vi "PH_HamamatsuCamera.PC Write PSDB.vi"(0 "i ref in":refnum<vi>, 5 "error IO":errorcluster) -> (14 "i ref out":refnum<vi>, 19 "error out":errorcluster)   [LabVIEW 2014, in "PH_HamamatsuCamera.lvlib"]
doc: "This is the proc case which writes data to the PHELIX shot data base."
uses:
  PH_HamamatsuCamera.lvlib
  PH_Basics/PH_PSDBWriter/PH_PSDBWriter.lvlib
  PH_Basics/PH_Cam_BaseClass/PH_Cam_BaseClass.lvlib
  PH_Basics/PH_StatusHandler/PH_StatusHandler.lvlib
panel:
  in  "Mode":u32(ring)=1 items=["Internal"=1, "External Edge"=2, "External Level"=4, "Software"=32, "Fast Repetition"=64, "TDI"=128, "Trigger Start"=512, "Sync Readout"=1024]
  in  "Polarity":u32(ring)=1 items=["Negative"=1, "Positive"=2]
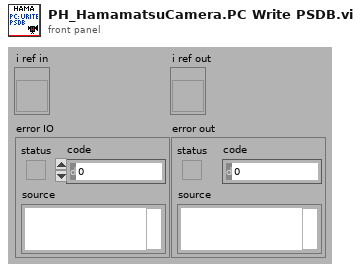
[diagram p1: front panel]
types:
  T1 = typedef "PH_HamamatsuCamera.lvlib/PH_HamamatsuCamera.i attribute.ctl" = cluster{"Gui Refs":cluster{"Camera Details":refnum<vi>, "ROI":refnum<vi>, "Set ROI to Maximum":refnum<vi>, "Trigger Parameters":refnum<vi>, "Brightness":refnum<vi>, "Shutter":refnum<vi>, "Gain":refnum<vi>, "Trigger Timeout":refnum<vi>, "Trigger Polarity":refnum<vi>, "Trigger Mode":refnum<vi>, "Parameters":refnum<vi>, "Set Cam Parameter":refnum<vi>, "Parameter to set":refnum<vi>, "Value to set":refnum<vi>}, "Cam":cluster{"Handle":i32, "Details":cluster{"Model":string, "Camera ID":string, "Firmware":string}, "Buffer Info":cluster{"height":u32, "width":u32, "datatype":u32}}, "H Offset":cluster{"Value":i32, "Minimum":i32, "Maximum":i32, "Increment":i32}, "V Offset":cluster{"Value":i32, "Minimum":i32, "Maximum":i32, "Increment":i32}, "H Width":cluster{"Value":i32, "Minimum":i32, "Maximum":i32, "Increment":i32}, "V Width":cluster{"Value":i32, "Minimum":i32, "Maximum":i32, "Increment":i32}, "Trigger Parameters":T2, "Trigger Timeout":u32, "Parameters":T3[], "Indicees Cam Parameters":cluster{"Brightness":i32, "Shutter":i32, "Gain":i32}, "Wanted Values":cluster{"Trigger Settings":T2[], "ROI":T4[], "Parameter":cluster{"Name":string, "Value":dbl}[]}}
  T2 = typedef "PH_HamamatsuCamera.lvlib/PH_HamamatsuCamera.Trigger Parameter.ctl" = cluster{"Mode":u32, "Polarity":u32, "Times":u32, "Delay":dbl}
  T3 = typedef "PH_HamamatsuCamera.lvlib/PH_HamamatsuCamera.Parameter Set.ctl" = cluster{"Parameter":string, "Value":dbl, "Writable":bool, "Range":cluster{"min":dbl, "max":dbl, "step":dbl}, "Default":dbl, "Value Names":cluster{"Name":string, "Value":dbl}[], "Text Values":bool}
  T4 = typedef "PH_HamamatsuCamera.lvlib/PH_HamamatsuCamera.ROI.ctl" = cluster{"Horizontal Offset":i32, "Vertical Offset":i32, "Horizontal Width":i32, "Vertical Width":i32}
  T5 = typedef "LVStringsAndValuesArrayTypeDef_U32.ctl" = cluster{"String":string, "Value":u32}[]
  T6 = typedef "PH_Cam_BaseClass.lvlib/PH_Cam_BaseClass.Settings.ctl" = cluster{"Cam ID":string, "Gain":dbl, "Brightness":dbl, "Shutter":dbl, "Mode":i32}
  T7 = typedef "PH_StatusHandler.lvlib/PH_StatusHandler.Status.ctl" = i16
  T8 = typedef "PH_Cam_BaseClass.lvlib/PH_Cam_BaseClass.i attribute.ctl" = cluster{"Gui Refs":T9, "Cam":cluster{"Source Notifier":refnum<notifier>, "Error":errorcluster, "Camera ID":string}, "Images":cluster{"Cam":T10, "Operation":T10, "PSDB":T10}, "Window Image":cluster{"Indicate Image":bool, "Window No.":i32, "Scale Facor":dbl, "Center Cross":bool, "Subtract Backgr":bool, "CoG":bool, "Color Palette":cluster{"Red":u8, "Green":u8, "Blue":u8}[], "Image On":bool}, "Default Prdc Int":i32, "Performance":cluster{"on":bool, "Timestamp Last Frame":i32}, "Histogram":cluster{"on":bool, "Mapping":bool}, "Save Image":cluster{"Save":bool, "File refnum":refnum<file>}, "Setting Service ID":i32, "Screen":cluster{"x-resolution":i16, "y-resolution":i16}, "On":bool, "Constructor finished":bool, "configured":bool}
  T9 = typedef "PH_Cam_BaseClass.lvlib/PH_Cam_BaseClass.GUI Refs.ctl" = cluster{"Frame Rate":refnum<vi>, "Get Frame Rate":refnum<vi>, "Show Image":refnum<vi>, "Get Histogram":refnum<vi>, "Mapping":refnum<vi>, "Histogram":refnum<vi>, "Center Cross":refnum<vi>, "Center of Gravity":refnum<vi>, "Scale Factor [%]":refnum<vi>, "Save Image":refnum<vi>, "Palette":refnum<vi>, "Subtract Background":refnum<vi>, "Cam Error":refnum<vi>, "On":refnum<vi>, "Cam List":refnum<vi>}
  T10 = typedef "IMAQ Image.ctl" = refnum<image>
  T11 = typedef "PH_PSDBWriter.lvlib/PH_PSDBWriter.Image dataset.ctl" = cluster{"name":string, "data":T10, "unit":string}
  T12 = typedef "PH_PSDBWriter.lvlib/PH_PSDBWriter.Numeric dataset.ctl" = cluster{"name":string, "data":dbl, "unit":string}
  T13 = typedef "PH_PSDBWriter.lvlib/PH_PSDBWriter.String dataset.ctl" = cluster{"name":string, "data":string, "unit":string}
  T14 = typedef "PH_PSDBWriter.lvlib/PH_PSDBWriter.PSDB Dataset.ctl" = cluster{"Version":i32, "2D data Input":T15[], "Boolean Input":T17[], "Image Input":T11[], "Numeric Input":T12[], "String Input":T13[]}
  T15 = typedef "PH_PSDBWriter.lvlib/PH_PSDBWriter.2D dataset.ctl" = cluster{"name":string, "data":dbl[][], "axis description":T16}
  T16 = typedef "PSDB.lvlib/PSDB_AxisDescription.ctl" = cluster{"x axis label":string, "y axis label":string, "x axis unit":string, "y axis unit":string}
  T17 = typedef "PH_PSDBWriter.lvlib/PH_PSDBWriter.Boolean dataset.ctl" = cluster{"name":string, "data":bool, "unit":string}
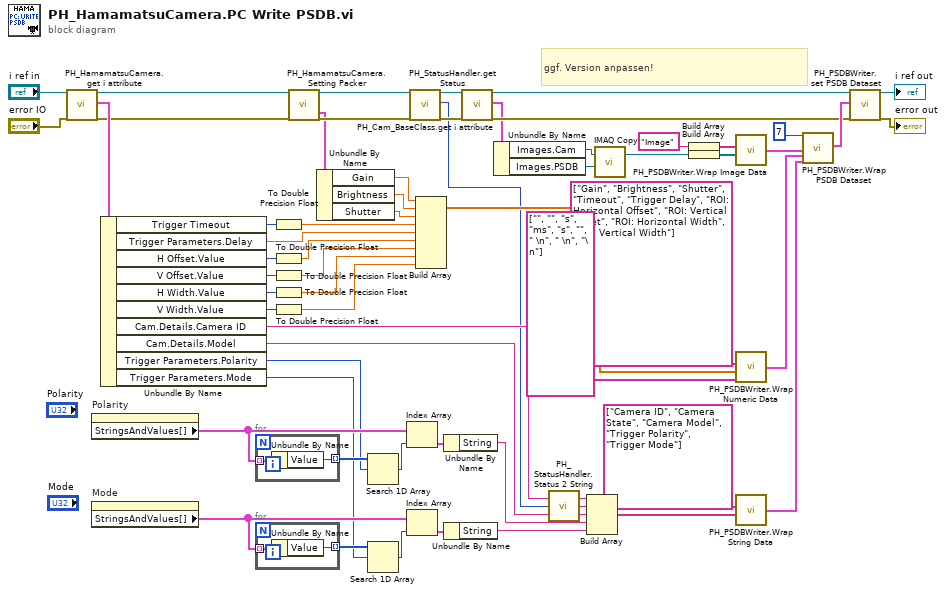
[diagram p0: block diagram]
diagram:
  # "ggf. Version anpassen!"
  n1 = call "PH_HamamatsuCamera.get i attribute.vi"("i ref in"="i ref in", "error in (no error)"="error IO") -> ("i ref out"=w38:refnum<vi>, "i attribute"=w57:T1, "error out"=w37:errorcluster)  [unwired: 15 in]
  n2 = property on="Polarity" class="Ring (strict)"() -> ("StringsAndValues[]"=w21:T5)  [unwired: 2 in, 2 out]
  n3 = property on="Mode" class="Ring (strict)"() -> ("StringsAndValues[]"=w15:T5)  [unwired: 2 in, 2 out]
  n4 = Unbundle By Name(w57) -> ("Trigger Timeout"=w58:u32, "Trigger Parameters.Delay"=w31:dbl, "H Offset.Value"=w12:i32, "V Offset.Value"=w11:i32, "H Width.Value"=w10:i32, "V Width.Value"=w9:i32, "Cam.Details.Camera ID"=w30:string, "Cam.Details.Model"=w55:string, "Trigger Parameters.Polarity"=w20:u32, "Trigger Parameters.Mode"=w14:u32)
  n5 = for {
    tunnel: w21 -> [w63] mode=indexing
    tunnel: [w62] -> w24 mode=indexing
    n6 = Unbundle By Name(w63) -> ("Value"=w62:u32)
  }
  n7 = for {
    tunnel: w15 -> [w65] mode=indexing
    tunnel: [w64] -> w18 mode=indexing
    n8 = Unbundle By Name(w65) -> ("Value"=w64:u32)
  }
  n9 = To Double Precision Float(number=w58) -> (double precision float=w59:dbl)
  n10 = To Double Precision Float(number=w12) -> (double precision float=w8:dbl)
  n11 = To Double Precision Float(number=w11) -> (double precision float=w7:dbl)
  n12 = To Double Precision Float(number=w10) -> (double precision float=w6:dbl)
  n13 = To Double Precision Float(number=w9) -> (double precision float=w5:dbl)
  n14 = call "PH_HamamatsuCamera.Setting Packer.vi"("i ref in"=w38, "error in (no error)"=w37) -> ("i ref out"=w3:refnum<vi>, "Cam Settings"=w35:T6, "error out"=w36:errorcluster)  [unwired: 15 in]
  n15 = Unbundle By Name(w35) -> ("Gain"=w34:dbl, "Brightness"=w33:dbl, "Shutter"=w32:dbl)
  n16 = Search 1D Array(1D array=w24, element=w20) -> (index of element=w23:i32)  [unwired: 1 in]
  n17 = Search 1D Array(1D array=w18, element=w14) -> (index of element=w17:i32)  [unwired: 1 in]
  n18 = Index Array(array=w21, index=w23) -> (element=w22:cluster{"String":string, "Value":u32})
  n19 = Index Array(array=w15, index=w17) -> (element=w16:cluster{"String":string, "Value":u32})
  n20 = call "PH_StatusHandler.get Status.vi"("VI in"=w3, "error in"=w36) -> ("VI out"=w2:refnum<vi>, "Status"=w1:T7, "error out"=w4:errorcluster)  [unwired: 15 in]
  n21 = Build Array(w34, w33, w32, w59, w31, w8, w7, w6, w5) -> (w47:dbl[])
  n22 = Unbundle By Name(w22) -> ("String"=w19:string)
  n23 = Unbundle By Name(w16) -> ("String"=w13:string)
  n24 = call "PH_Cam_BaseClass.get i attribute.vi"("i ref in"=w2, "error in (no error)"=w4) -> ("i ref out"=w28:refnum<vi>, "i attribute"=w27:T8, "error out"=w29:errorcluster)  [unwired: 15 in]
  n25 = Unbundle By Name(w27) -> ("Images.Cam"=w26:T10, "Images.PSDB"=w25:T10)
  n26 = call "PH_StatusHandler.Status 2 String.vi"("Status"=w1) -> ("Status as string"=w56:string)
  n27 = Build Array(w30, w56, w55, w19, w13) -> (w52:string[])
  n28 = call "IMAQ Copy"("Image Dst"=w25, "Image Src"=w26) -> ("Image Dst Out"=w42:T10)  [unwired: 4 in, 1 out]
  n29 = Build Array("Image" ("name")) -> (w39:string[])
  n30 = Build Array(w42) -> (w41:T10[])
  n31 = call "PH_PSDBWriter.Wrap Image Data.vi"("Data Arrray"=w41, "Name Array"=w39) -> ("PSDB Image Data Array"=w44:T11[])  [unwired: 2 in]
  n32 = call "PH_PSDBWriter.Wrap Numeric Data.vi"("Unit Array"=string[] ["", "", "s", "ms", "s", "", " \n", " \n", "\n"], "Data Array"=w47, "Name Array"=string[] ["Gain", "Brightness", "Shutter", "Timeout", "Trigger Delay", "ROI: Horizontal Offset", "ROI: Vertical Offset", "ROI: Horizontal Width", "ROI: Vertical Width"]) -> ("PSDB Numeric Data Array"=w45:T12[])  [unwired: 1 in]
  n33 = call "PH_PSDBWriter.Wrap String Data.vi"("Data Array"=w52, "Name Array"=string[] ["Camera ID", "Camera State", "Camera Model", "Trigger Polarity", "Trigger Mode"]) -> ("PSDB String Data Array"=w51:T13[])  [unwired: 2 in]
  n34 = call "PH_PSDBWriter.Wrap PSDB Dataset.vi"("Version"=7, "Image Input"=w44, "Numeric Input"=w45, "String Input"=w51) -> ("PSDB Dataset"=w50:T14)  [unwired: 15 in]
  n35 = call "PH_PSDBWriter.set PSDB Dataset.vi"("VI in"=w28, "PSDB Dataset"=w50, "error in (no error)"=w29) -> ("VI out"=→"i ref out":refnum<vi>, "error out"=→"error out":errorcluster)  [unwired: 15 in]
